vi "Write Meta Values.vi"(8 "error in (no error)":errorcluster, 10 "Meta Data":T1[](array[typedef]), 11 "Config Element in":refnum<class "Config Element.lvclass">) -> (0 "error out":errorcluster, 3 "Config Element out":refnum<class "Config Element.lvclass">)   [LabVIEW 2023, in "CDM-Config.lvlib" / "Config Element.lvclass"]
doc: "Writes multiple meta values to the element. Any existing meta values with the same name will have their value overwritten with the new specified value."
uses:
  Config Element.lvclass
  Meta Data.ctl
  Config Element.lvclass/Config Element.ctl
  CDM-Config.lvlib
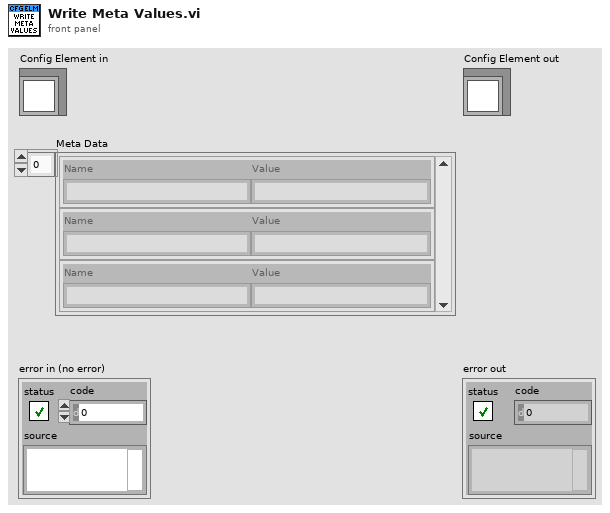
[diagram p1: front panel]
types:
  T1 = typedef "CDM-Config.lvlib/Meta Data.ctl" = cluster{"Name":string, "Value":string}
  T2 = typedef "CDM-Config.lvlib/Config Element.lvclass/Element Data.ctl" = cluster{"Node Info":T3, "Owner":refnum<class>, "Changed":bool, "Name":string, "Meta Data":T1[], "Value Type":T4, "Value":variant}
  T3 = typedef "CDM-Config.lvlib/Node Info.ctl" = cluster{"Index":i32, "Parent":i32, "Children":i32[]}
  T4 = typedef "CDM-Config.lvlib/Value Type.ctl" = enum16{"String", "Number", "Bool", "Object", "Array"}
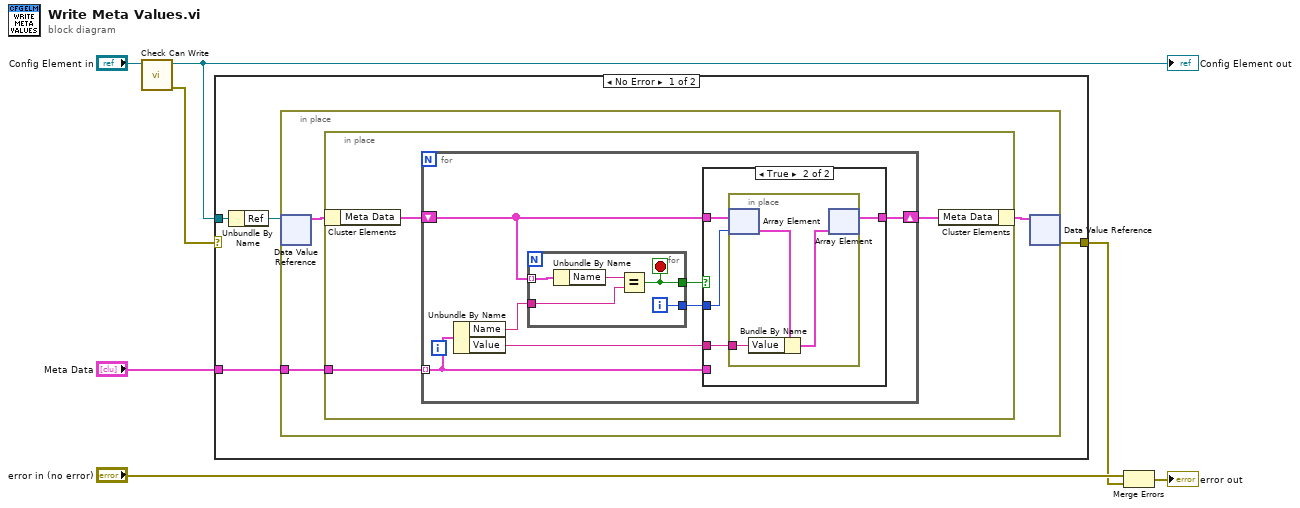
[diagram p0: block diagram]
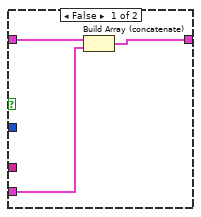
[diagram p2: hidden frame]
diagram:
  n1 = call "Check Can Write.vi"("Config Element in"="Config Element in") -> ("error out"=w1:errorcluster, "Config Element out"=w2:refnum<class "Config Element.lvclass">)  [unwired: 9 in]
  "Config Element out" <- w2
  n2 = case shown="No Error" w1 {
    selector: w1 -> [_ w40]
    tunnel: "Meta Data" -> [w10 _]
    tunnel: [w9 w40] -> w3
    tunnel: w2 -> [w8 _]
    frame No Error {
      n3 = Unbundle By Name(w8) -> ("Ref"=w11:refnum<data-value>)
      n4 = in-place {
        in-place-border: w10 -> [w12]
        n5 = in-place-dvr #1(w11) -> (w14:T2)  [unwired: 1 out]
        n6 = in-place {
          in-place-border: w12 -> [w16]
          n7 = in-place-cluster #2(w14) -> ("Meta Data"=w17:T1[])
          n8 = for {
            shift-right: [w19] -> w15
            shift-left: w17 -> [w21]
            tunnel: w16 -> [w18] mode=indexing
            n9 = Unbundle By Name(w18) -> ("Name"=w24:string, "Value"=w20:string)
            n10 = for {
              tunnel: w21 -> [w39] mode=indexing
              tunnel: w24 -> [w37]
              tunnel: [w36] -> w23
              tunnel: [w35] -> w22
              i -> [w35]
              stop <- w36 stop-if-true
              n11 = Unbundle By Name(w39) -> ("Name"=w38:string)
              n12 = Equal?(x=w38, y=w37) -> (x = y?=w36:bool)
            }
            n13 = case shown="True" w23 {
              tunnel: w22 -> [_ w29]
              tunnel: w21 -> [w27 w30]
              tunnel: w20 -> [_ w31]
              tunnel: [w25 w28] -> w19
              tunnel: w18 -> [w26 _]
              frame False {
                n14 = Build Array (concatenate)(w27, w26) -> (w25:T1[])
              }
              frame True {
                n15 = in-place {
                  in-place-border: w31 -> [w33]
                  n16 = in-place-array #3(w30, w29) -> (w34:T1)
                  n17 = Bundle By Name(cluster=w34, "Value"=w33) -> (w32:T1)
                  n18 = in-place-array #3(w32) -> (w28:T1[])  [unwired: 1 out]
                }
              }
            }
          }
          n19 = in-place-cluster #2("Meta Data"=w15) -> (w13:T2)
        }
        n20 = in-place-dvr #1(w13) -> (w9:errorcluster)  [unwired: 1 out]
      }
    }
    frame Error {
    }
  }
  n21 = Merge Errors("error in (no error)", w3) -> (→"error out":errorcluster)
